vi "RUN.vi"(0 "VISA resource name":refnum<visa-resource-name>, 5 "Run Query":bool=TRUE, 11 "error in (no error)":errorcluster) -> (4 "VISA resource name out":refnum<visa-resource-name>, 6 "RUN":bool, 8 "Error Message":string, 10 "Error Code":i32, 15 "error out":errorcluster)   [LabVIEW 2010, in "VITREK V7X.lvlib"]
doc: "Runs the active test sequence if Run Query is No. RUN indicator is always False in this case.\n\nResponds with a <BOOL> indicating if the active test sequence is being run (1) or not (0), if Run Query is Yes.\n\n<b>Note:</b> please refer to the instrument manual for the <b>RUN(?)</b> specification."
uses:
  VITREK V7X.lvlib
panel:
  # "Yes\n\nNo"
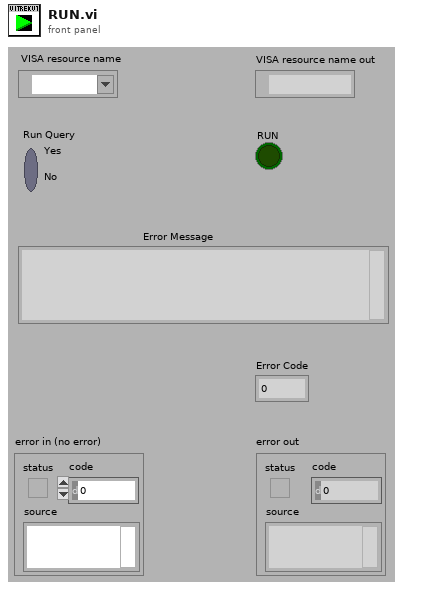
[diagram p1: front panel]
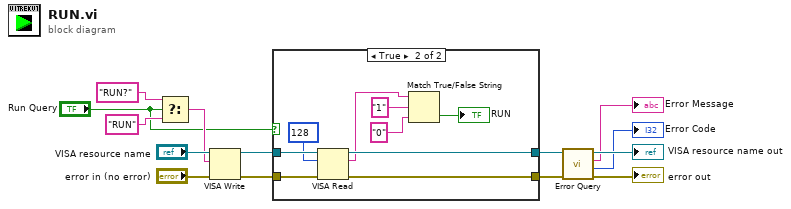
[diagram p0: block diagram]
diagram:
  n1 = Select(t="RUN?", s="Run Query", f="RUN" ("LOCKOUT Command")) -> (s? t:f=w8:string)
  n2 = VISA Write(VISA resource name="VISA resource name", write buffer=w8, error in (no error)="error in (no error)") -> (VISA resource name out=w6:refnum<visa-resource-name>, error out=w4:errorcluster)  [unwired: 1 out]
  n3 = case shown="True" "Run Query" {
    tunnel: w6 -> [w16 w24]
    tunnel: [w16 w22] -> w5
    tunnel: w4 -> [w15 w25]
    tunnel: [w15 w21] -> w3
    frame False {
    }
    frame True {
      n4 = VISA Read(VISA resource name=w24, byte count=u32 128, error in (no error)=w25) -> (VISA resource name out=w22:refnum<visa-resource-name>, read buffer=w19:string, error out=w21:errorcluster)  [unwired: 1 out]
      n5 = Match True/False String(2:"0", 3:"1", 4:w19) -> (0:→"RUN":bool)  [unwired: 1 out]
    }
  }
  n6 = call "Error Query.vi"("error in (no error)"=w3, "VISA resource name"=w5) -> ("error out"=→"error out":errorcluster, "Error Code"=→"Error Code":i32, "Error Message"=→"Error Message":string, "VISA resource name out"=→"VISA resource name out":refnum<visa-resource-name>)  [unwired: 6 in]
